vi "DFD FXP LabVIEW FPGA Code Generator.vi"(5 "open project? (F)":bool, 6 "confirm? (T)":bool=TRUE, 7 "# channels":i32=1, 8 "error in (no error)":errorcluster, 9 "filter name":string, 10 "destination folder":path, 11 "filter in":T1={"mSRate_Fs"=1.0, "mSRate_Version"="2.0", "mSRate_Comments"="", "mSRate_OrgCoef"={"type"=enum."Undefined", "gain"=1.0, "coef a (k)"=[], "coef b (v)"=[]}, "mSRate_CurCoef"={"type"=enum."Undefined", "gain"=1.0, "coef a (k)"=[], "coef b (v)"=[]}, "mSRate_Quantized?"=FALSE, "mSRate_QCoef"={"type"=enum."Undefined", "gain"=1.0, "coef a (k)"=[], "coef b (v)"=[]}, "mSRate_QSettings"=[], "mSRate_Order"=0, "mSRate_Scaling"={"mSRate_ScaleByPowerOf2?"=FALSE, "mSRate_ScaleType"=enum."No Norm"}} {"mSRate_QSettings"."source" items=["Coef a/k"=0, "Coef b/v"=7, "Input"=1, "Output"=2, "Multiplicand"=3, "Product"=4, "Sum"=5, "Delay"=6, "Gain"=8]}) -> (0 "error out":errorcluster, 1 "sampling frequency/FPGA clock":dbl, 2 "lvproj path":path)   [LabVIEW 2017, in "NI_DigFilterLicensed.lvlib"]
doc: "Generates fixed-point code from a fixed-point filter, including fixed-point LabVIEW field-programmable gate array (FPGA) code, integer LabVIEW code, and C code. You must manually select the polymorphic instance you want to use."
uses:
  <vilib>/addons/Digital Filter Design/NI_DigFilterLicensed.lvlib
  <vilib>/addons/Digital Filter Design/_Objects.llb/DFD Filter Obj.ctl
  <vilib>/addons/Digital Filter Design/_Objects.llb/DFD Filter Coef.ctl
  <vilib>/addons/Digital Filter Design/_Objects.llb/DFD Filter Structure Type Selector.ctl
  <vilib>/addons/Digital Filter Design/_Objects.llb/dfd_Internal Quantization Settings.ctl
  <vilib>/addons/Digital Filter Design/_Objects.llb/dfd_Internal Quantization Srcs.ctl
  <vilib>/addons/Digital Filter Design/_Objects.llb/DFD Coef Norm Type.ctl
  <vilib>/addons/Digital Filter Design/nMAC.llb/Typedefs/dfd_nMAC_Parameter.ctl
  <vilib>/addons/Digital Filter Design/nMAC.llb/Typedefs/dfd_nMAC_Memory Type.ctl
  <vilib>/addons/Digital Filter Design/nMAC.llb/Typedefs/dfd_nMAC_Coef Reload API.ctl
  <vilib>/addons/Digital Filter Design/nMAC.llb/Typedefs/dfd_nMAC_Execution Mode.ctl
  <vilib>/addons/Digital Filter Design/NI_DigFilter_CodeGen.lvlib
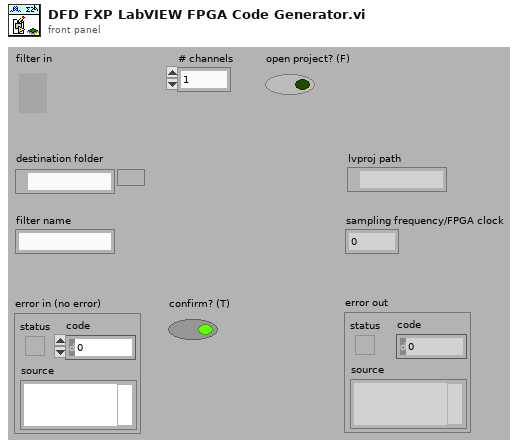
[diagram p1: front panel]
types:
  T1 = typedef "NI_DigFilterLicensed.lvlib/DFD Filter Obj.ctl" = cluster{"mSRate_Fs":dbl, "mSRate_Version":string, "mSRate_Comments":string, "mSRate_OrgCoef":T2, "mSRate_CurCoef":T2, "mSRate_Quantized?":bool, "mSRate_QCoef":T2, "mSRate_QSettings":T4[], "mSRate_Order":i32, "mSRate_Scaling":cluster{"mSRate_ScaleByPowerOf2?":bool, "mSRate_ScaleType":T6}}
  T2 = typedef "NI_DigFilterLicensed.lvlib/DFD Filter Coef.ctl" = cluster{"type":T3, "gain":dbl, "coef a (k)":dbl[], "coef b (v)":dbl[]}
  T3 = typedef "NI_DigFilterLicensed.lvlib/DFD Filter Structure Type Selector.ctl" = enum16{"Undefined", "FIR Direct Form", "FIR Direct Form Transposed", "FIR Symmetric", "FIR Antisymmetric", "IIR Direct Form I", "IIR Direct Form I Transposed", "IIR Direct Form II", "IIR Direct Form II Transposed", "IIR Cascaded Second Order Sections Form I", "IIR Cascaded Second Order Sections Form I Transposed", "IIR Cascaded Second Order Sections Form II", "IIR Cascaded Second Order Sections Form II Transposed", "Lattice Allpass (basic sections)", "Lattice Allpass (one multiplier sections)", "Lattice Allpass (normalized sections)", "Lattice AR (basic sections)", "Lattice AR (one multiplier sections)", "Lattice AR (normalized sections)", "Lattice MA (minimum phase)", "Lattice MA (maximum phase)", "Lattice ARMA (basic sections)", "Lattice ARMA (one multiplier sections)", "Lattice ARMA (normalized sections)"}
  T4 = typedef "NI_DigFilterLicensed.lvlib/dfd_Internal Quantization Settings.ctl" = cluster{"source":T5, "wl":i16, "iwl":i16, "overflow mode":enum16{"Saturation", "Wrap"}, "rounding mode":enum16{"Nearest", "Truncation"}, "signed?":bool}
  T5 = typedef "NI_DigFilterLicensed.lvlib/dfd_Internal Quantization Srcs.ctl" = u16
  T6 = typedef "NI_DigFilterLicensed.lvlib/DFD Coef Norm Type.ctl" = enum16{"No Norm", "Time Domain 1-Norm", "Time Domain 2-Norm", "Time Domain Inf-Norm"}
  T7 = typedef "dfd_nMAC_Execution Mode.ctl" = enum16{"Outside SCTL", "Inside SCTL"}
  T8 = typedef "dfd_nMAC_Parameter.ctl" = cluster{"#MACs":u32, "#level per register":u32, "#multiply pipeline stage":u32, "multiply register in":bool, "#paths":u32, "state memory":T9, "coefficient memory":T9, "coefficient reloadable":bool, "coefficient reload API":T10}
  T9 = typedef "dfd_nMAC_Memory Type.ctl" = enum16{"Automatic", "BRAM", "DRAM"}
  T10 = typedef "dfd_nMAC_Coef Reload API.ctl" = enum16{"Multiple interfaces", "Single interface"}
  T11 = typedef "dfd_nMAC_Implementation Parameter.ctl" = cluster{"common parameters":cluster{"execution mode":T7, "number of channels":u32, "reset":bool, "include overflow status":bool, "4-wire":bool}, "specific parameters":cluster{"number of MACs":u32, "multiply pipeline stages":u32, "multiply register in":bool, "#level per register":u32, "state memory":T9, "coefficient memory":T9, "number of paths":u32, "coefficient reloadable":bool, "coefficient reload API":T10, "coef map type":T12, "set vs channel map":u32[]}}
  T12 = typedef "dfd_nMAC_Coef Map Type.ctl" = enum16{"No Map", "Set Map", "Channel Map"}
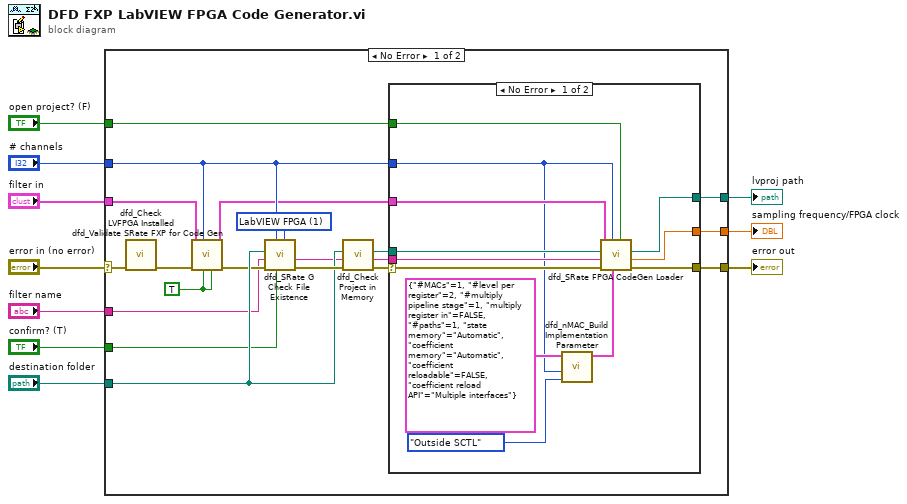
[diagram p0: block diagram]
diagram:
  n1 = case shown="No Error" "error in (no error)" {
    selector: "error in (no error)" -> [w12 w44]
    tunnel: [w27 _] -> w10
    tunnel: [w26 w44] -> w9
    tunnel: [w25 _] -> w8
    tunnel: "destination folder" -> [w23 _]
    tunnel: "# channels" -> [w22 _]
    tunnel: "confirm? (T)" -> [w21 _]
    tunnel: "open project? (F)" -> [w19 _]
    tunnel: "filter in" -> [w15 _]
    tunnel: "filter name" -> [w14 _]
    frame No Error {
      w20 = u16 1 items=["Integer LabVIEW", "LabVIEW FPGA"] ("code type")
      w30 = TRUE ("LabVIEW?")
      n2 = call <vilib>:"dfd_Check LVFPGA Installed.vi"("error in (no error)"=w12) -> ("error out"=w17:errorcluster)  [unwired: 10 out]
      n3 = call <vilib>:"dfd_Validate SRate FXP for Code Gen.vi"("FPGA?"=w30, "LabVIEW?"=w30, "totalChan"=w22, "error in"=w17, "filter"=w15) -> ("error out"=w16:errorcluster, "dup filter"=w11:T1)  [unwired: 5 out]
      n4 = call <vilib>:"dfd_SRate G Check File Existence.vi"("code type"=w20, "confirm?"=w21, "# channels"=w22, "error in (no error)"=w16, "filter name"=w14, "dest path"=w23) -> ("error out"=w24:errorcluster, "filter name out"=w13:string)  [unwired: 1 in, 3 out]
      n5 = call <vilib>:"dfd_Check Project in Memory.vi"("error in (no error)"=w24, "filter name"=w13, "dest path"=w23) -> ("error out"=w18:errorcluster, "filter name out"=w28:string, "dup dest path"=w29:path)  [unwired: 6 out]
      n6 = case shown="No Error" w18 {
        selector: w18 -> [w40 w43]
        tunnel: w11 -> [w35 _]
        tunnel: w29 -> [w42 _]
        tunnel: w28 -> [w41 _]
        tunnel: w22 -> [w32 _]
        tunnel: [w39 _] -> w27
        tunnel: [w38 w43] -> w26
        tunnel: [w37 _] -> w25
        tunnel: w19 -> [w36 _]
        frame No Error {
          n7 = call <vilib>:"dfd_nMAC_Build Implementation Parameter.vi"("execution mode"=dfd_nMAC_Execution_Mode."Outside SCTL", "# channels"=w32, "nMAC Parameters"=T8 {"#MACs"=1, "#level per register"=2, "#multiply pipeline stage"=1, "multiply register in"=FALSE, "#paths"=1, "state memory"=enum."Automatic", "coefficient memory"=enum."Automatic", "coefficient reloadable"=FALSE, "coefficient reload API"=enum."Multiple interfaces"}) -> ("implementation para in"=w33:T11)  [unwired: 8 in]
          n8 = call <vilib>:"dfd_SRate FPGA CodeGen Loader.vi"("open project? (F)"=w36, "implementation para in"=w33, "# channels"=w32, "error in (no error)"=w40, "filter name"=w41, "destination path"=w42, "filter in"=w35) -> ("error out"=w38:errorcluster, "sampling rate/FPGA clock"=w39:dbl, "lvproj path"=w37:path)  [unwired: 2 out]
        }
        frame Error {
        }
      }
    }
    frame Error {
    }
  }
  "error out" <- w9
  "sampling frequency/FPGA clock" <- w10
  "lvproj path" <- w8
